vi "Remove Constant Current 1.vi"(3 "error in":errorcluster) -> (10 "error out":errorcluster)   [LabVIEW 2015]
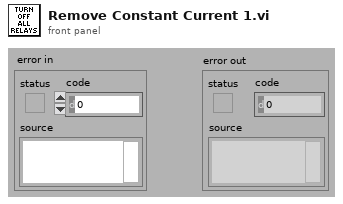
[diagram p1: front panel]
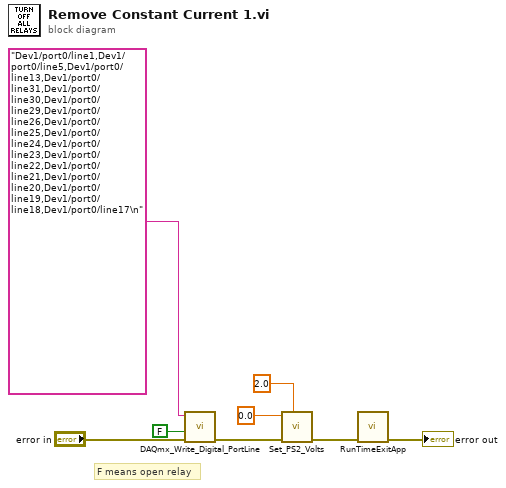
[diagram p0: block diagram]
diagram:
  # "F means open relay"
  n1 = call "DAQmx_Write_Digital_PortLine.vi"("Device/Ports/Lines"="Dev1/port0/line1,Dev1/port0/line5,Dev1/port0/line13,Dev1/port0/line31,Dev1/port0/line30,Dev1/port0/line29,Dev1/port0/line26,Dev1/port0/line25,Dev1/port0/line24,Dev1/port0/line23,Dev1/port0/line22,Dev1/port0/line21,Dev1/port0/line20,Dev1/port0/line19,Dev1/port0/line18,Dev1/port0/line17\n", "Boolean"=FALSE, "error in"="error in") -> ("error out"=w5:errorcluster)  [unwired: 6 in, 1 out]
  n2 = call "Set_PS2_Volts.vi"("Output Voltage"=0.0 ("Output Voltage (0)"), "error in"=w5, "delay (secs)"=2.0) -> ("error out"=w4:errorcluster)  [unwired: 5 in, 2 out]
  n3 = call "RunTimeExitApp.vi"("error in (no error)"=w4) -> ("error out"=→"error out":errorcluster)  [unwired: 10 in]
